vi "Delete_Crossconnection-2.vi"(5 "[IN] Row index\nInitial Point":i32, 7 "[IN] Column in\ndex Initial Point":i32, 9 "[IN] Indicies of Cross\nconnected Points":i32[](array[numeric]), 10 "[IN] The other point \nfor crossconnection found":bool, 11 "[IN] Track group":T1) -> (1 "[OUT] Track group":T1, 2 "[OUT] Column index\nCorrect initial point":i32, 3 "[OUT] Row index\nCorrect initial point":i32)   [LabVIEW 2017]
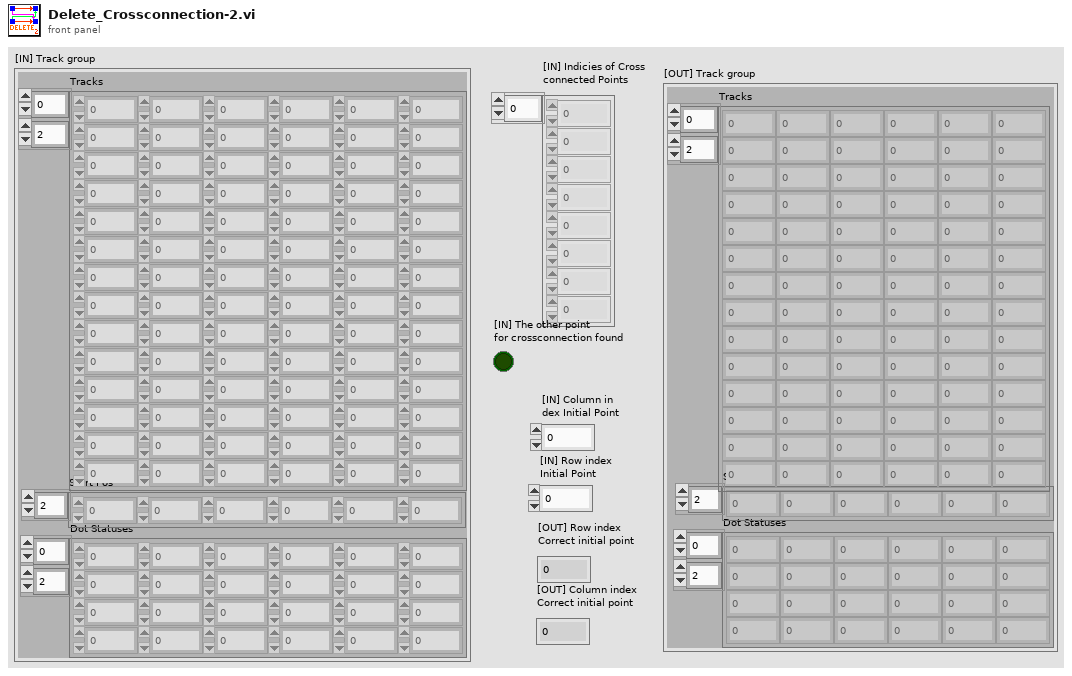
[diagram p1: front panel]
types:
  T1 = cluster{"Tracks":dbl[][], "Start Pos":i32[], "Dot Statuses":i16[][]}
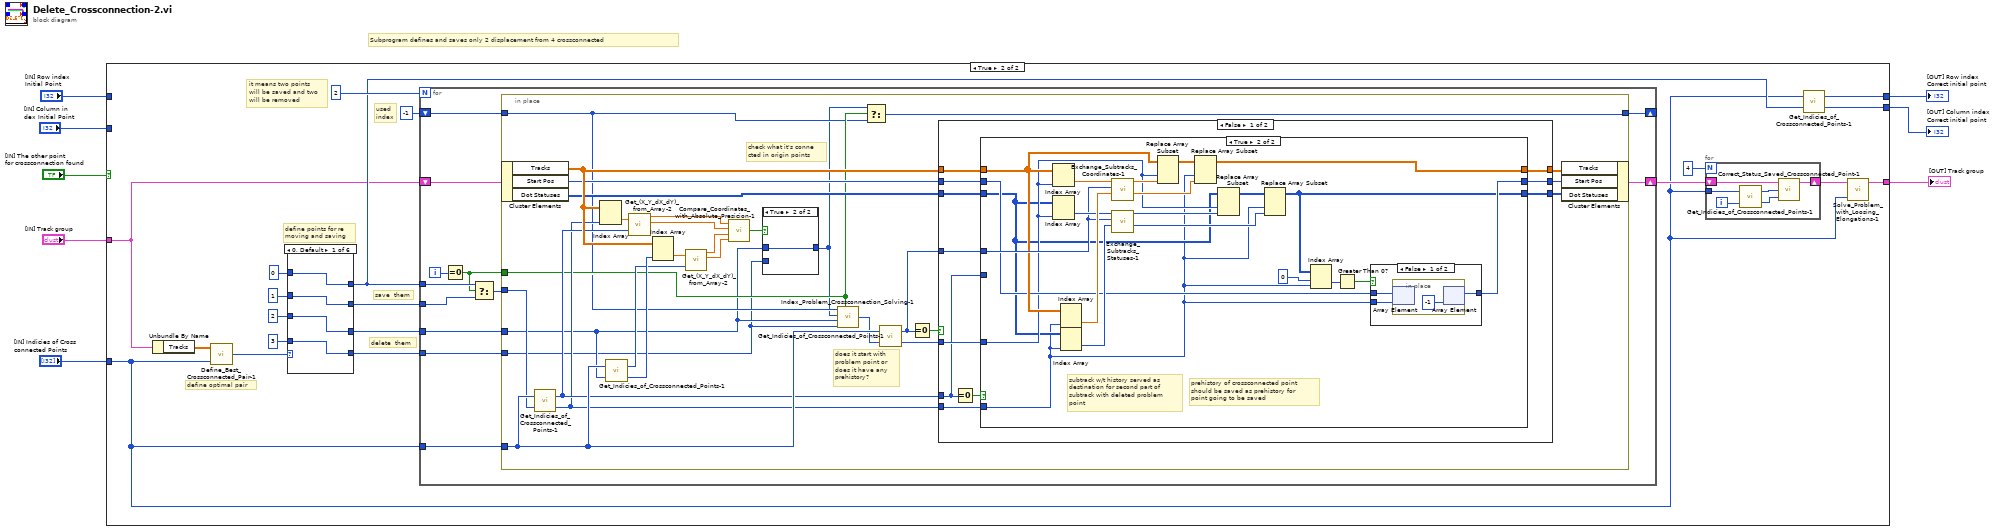
[diagram p0: block diagram]
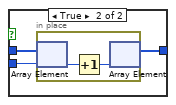
[diagram p4: hidden frame]
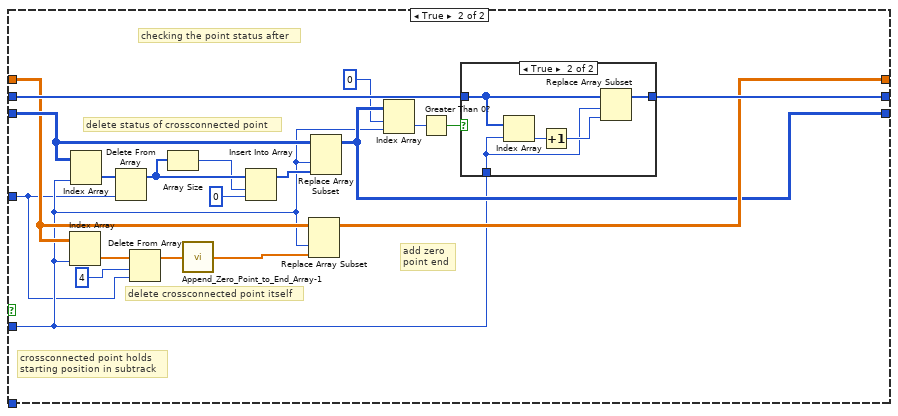
[diagram p5: hidden frame]
diagram:
  # "Subprogram defines and saves only 2 displacement from 4 crossconnected"
  n1 = case shown="True" "[IN] The other point \nfor crossconnection found" {
    tunnel: "[IN] Track group" -> [w11 w19]
    tunnel: "[IN] Indicies of Cross\nconnected Points" -> [_ w13]
    tunnel: [w11 w12] -> w5
    tunnel: [w10 w22] -> w4
    tunnel: [w9 w21] -> w3
    tunnel: "[IN] Row index\nInitial Point" -> [w10 _]
    tunnel: "[IN] Column in\ndex Initial Point" -> [w9 _]
    frame False {
    }
    frame True {
      # "define optimal pair"
      # "used \nindex"
      # "it means two points\nwill be saved and two\nwill be removed"
      # "define points for re\nmoving and saving"
      # "delete  them"
      # "save  them"
      n2 = Unbundle By Name(w19) -> ("Tracks"=w18:dbl[][])
      n3 = call "Define_Best_Crossconnected_Pair-1.vi"("[IN] Indicies of Cross\nconnected Points"=w13, "[IN] Tracks"=w18) -> ("[OUT] Smallest Pair"=w17:i32)  [unwired: 3 in]
      n4 = case shown="0, Default" w17 {
        tunnel: 0 -> [w155 w159 w163 w165 w169 w173]
        tunnel: 1 -> [w154 w157 w161 w167 w171 w172]
        tunnel: 2 -> [w153 w158 w160 w166 w168 w175]
        tunnel: 3 -> [w152 w156 w162 w164 w170 w174]
        tunnel: [w155 w159 w163 w167 w171 w175] -> w23
        tunnel: [w154 w158 w162 w166 w170 w174] -> w24
        tunnel: [w153 w157 w161 w165 w169 w173] -> w27
        tunnel: [w152 w156 w160 w164 w168 w172] -> w26
        frame 0, Default {
        }
        frame 1 {
        }
        frame 2 {
        }
        frame 3 {
        }
        frame 4 {
        }
        frame 5 {
        }
      }
      n5 = for {
        N: 2 -> [_]
        tunnel: w13 -> [w48]
        tunnel: w23 -> [w43]
        tunnel: w24 -> [w42]
        tunnel: w27 -> [w47]
        tunnel: w26 -> [w46]
        shift-right: [w45] -> w15
        shift-left: w19 -> [w49]
        shift-right: [w39] -> _
        shift-left: -1 -> [w40]
        i -> [w44]
        n6 = Equal To 0?(x=w44) -> (x = 0?=w38:bool)
        n7 = Select(t=w43, s=w38, f=w42) -> (s? t:f=w41:i32)
        n8 = in-place {
          in-place-border: w48 -> [w69]
          in-place-border: w47 -> [w51]
          in-place-border: w46 -> [w50]
          in-place-border: w41 -> [w59]
          in-place-border: w40 -> [w54]
          in-place-border: [w56] -> w39
          in-place-border: w38 -> [w55]
          # "does it start with \nproblem point or\ndoes it have any \nprehistory?"
          # "check what it's conne\ncted in origin points"
          n9 = in-place-cluster #1(w49) -> ("Tracks"=w67:dbl[][], "Start Pos"=w66:i32[], "Dot Statuses"=w65:i16[][])
          n10 = call "Get_Indicies_of_Crossconnected_Points-1.vi"("[IN] Index of point"=w59, "[IN] Indicies of Cross\nconnected Points"=w69) -> ("[OUT] Column index"=w57:i32, "[OUT] Row index"=w58:i32)
          n11 = Index Array(array=w67, index (col)=w57) -> (element=w78:dbl[])  [unwired: 1 in]
          n12 = call "Get_Indicies_of_Crossconnected_Points-1.vi"("[IN] Index of point"=w51, "[IN] Indicies of Cross\nconnected Points"=w69) -> ("[OUT] Column index"=w77:i32, "[OUT] Row index"=w75:i32)
          n13 = call "Get_(X_Y_dX_dY)_from_Array-2.vi"("(X,Y,dX,dY)"=w78, "Index of Displacement"=w58) -> ("X"=w74:dbl, "Y"=w73:dbl)  [unwired: 2 out]
          n14 = Index Array(array=w67, index (col)=w77) -> (element=w76:dbl[])  [unwired: 1 in]
          n15 = call "Get_(X_Y_dX_dY)_from_Array-2.vi"("(X,Y,dX,dY)"=w76, "Index of Displacement"=w75) -> ("X"=w72:dbl, "Y"=w71:dbl)  [unwired: 2 out]
          n16 = call "Compare_Coordinates_with_Absolute_Presicion-1.vi"("X 1"=w74, "Y 1"=w73, "X 2"=w72, "Y 2"=w71) -> ("[OUT] Same coordinates?"=w70:bool)  [unwired: 1 in]
          n17 = case shown="True" w70 {
            tunnel: w51 -> [_ w151]
            tunnel: w50 -> [w150 _]
            tunnel: [w150 w151] -> w53
            frame False {
            }
            frame True {
            }
          }
          n18 = call "Index_Problem_Crossconnection_Solving-1.vi"("[IN] Used Index"=w54, "[IN] Defined Index"=w53, "[IN] 1st Index for Deletion"=w51, "[IN] 2nd Index for Deletion"=w50, "[IN] Is it first step?"=w55) -> ("[OUT] Index of Track wi\nth Point For Deletion"=w52:i32)
          n19 = Select(t=w53, s=w55, f=w54) -> (s? t:f=w56:i32)
          n20 = call "Get_Indicies_of_Crossconnected_Points-1.vi"("[IN] Index of point"=w52, "[IN] Indicies of Cross\nconnected Points"=w69) -> ("[OUT] Column index"=w64:i32, "[OUT] Row index"=w62:i32)
          n21 = Equal To 0?(x=w62) -> (x = 0?=w68:bool)
          n22 = case shown="False" w68 {
            tunnel: w67 -> [w88 w133]
            tunnel: w66 -> [w87 w143]
            tunnel: w65 -> [w86 w138]
            tunnel: w64 -> [w81 w128]
            tunnel: [w84 w142] -> w63
            tunnel: w62 -> [w80 w125]
            tunnel: [w85 w131] -> w61
            tunnel: [w83 w129] -> w60
            tunnel: w58 -> [w79 _]
            tunnel: w57 -> [w82 _]
            frame False {
              n23 = Equal To 0?(x=w79) -> (x = 0?=w89:bool)
              n24 = case shown="True" w89 {
                tunnel: w88 -> [w92 w109]
                tunnel: w87 -> [w91 w100]
                tunnel: w86 -> [w90 w97]
                tunnel: [w92 w105] -> w85
                tunnel: [w91 w98] -> w84
                tunnel: [w90 w96] -> w83
                tunnel: w82 -> [_ w95]
                tunnel: w81 -> [_ w99]
                tunnel: w80 -> [_ w110]
                tunnel: w79 -> [_ _]
                frame False {
                  # "I suppose that tracking algorithm will be able to resolve such problem in this case"
                }
                frame True {
                  # "subtrack w/t history served as \ndestination for second part of \nsubtrack with deleted problem \npoint"
                  # "prehistory of crossconnected point \nshould be saved as prehistory for \npoint going to be saved"
                  n25 = Index Array(array=w109, index (col)=w99) -> (element=w114:dbl[])  [unwired: 1 in]
                  n26 = Index Array(array=w97, index (col)=w99) -> (element=w112:i16[])  [unwired: 1 in]
                  n27 = Index Array(array=w109, index (col)=w95) -> (element=w113:dbl[])  [unwired: 1 in]
                  n28 = Index Array(array=w97, index (col)=w95) -> (element=w111:i16[])  [unwired: 1 in]
                  n29 = call "Exchange_Subtracks_Coordinates-1.vi"("[IN] Subtrack wit\nhout prehistory"=w113, "[IN] Row index \nProblem Point"=w110, "[IN] Subtrack \nwith problem"=w114) -> ("[OUT] Reconnected subtrack\n(posthistory after deleted \ncrossconnected point)"=w106:dbl[], "[OUT] Reconnected subtrack\nPrehistory + alternative prob\nlem point"=w108:dbl[])  [unwired: 3 in]
                  n30 = call "Exchange_Subtracks_Statuses-1.vi"("[IN] Statuses wit\nhout prehistory"=w111, "[IN] Row index \nProblem Point"=w110, "[IN] Statuses\nwith problem"=w112) -> ("[OUT] Reconnected statuses\n(posthistory after deleted \ncrossconnected point)"=w102:i16[], "[OUT] Reconnected statuses\nPrehistory + alternative prob\nlem point"=w104:i16[])  [unwired: 3 in]
                  n31 = Replace Array Subset(array=w109, new element=w108, index (col)=w99) -> (w107:dbl[][])  [unwired: 1 in]
                  n32 = Replace Array Subset(array=w107, new element=w106, index (col)=w95) -> (w105:dbl[][])  [unwired: 1 in]
                  n33 = Replace Array Subset(array=w97, new element=w104, index (col)=w99) -> (w103:i16[][])  [unwired: 1 in]
                  n34 = Replace Array Subset(array=w103, new element=w102, index (col)=w95) -> (w96:i16[][])  [unwired: 1 in]
                  n35 = Index Array(array=w96, index (row)=0 ("disabled index (row)"), index (col)=w95) -> (element=w101:i16)
                  n36 = Greater Than 0?(x=w101) -> (x > 0?=w93:bool)
                  n37 = case shown="False" w93 {
                    tunnel: w100 -> [w117 w121]
                    tunnel: w95 -> [w116 w120]
                    tunnel: [w115 w119] -> w98
                    frame False {
                      n38 = in-place {
                        n39 = in-place-array #2(w117, w116) -> ()  [unwired: 1 out]
                        n40 = in-place-array #2(-1) -> (w115:i32[])  [unwired: 1 out]
                      }
                    }
                    frame True {
                      n41 = in-place {
                        n42 = in-place-array #3(w121, w120) -> (w123:i32)
                        n43 = Increment(x=w123) -> (x+1=w122:i32)
                        n44 = in-place-array #3(w122) -> (w119:i32[])  [unwired: 1 out]
                      }
                    }
                  }
                }
              }
            }
            frame True {
              # "add zero \npoint end"
              # "checking the point status after"
              # "delete crossconnected point itself"
              # "delete status of crossconnected point"
              # "crossconnected point holds \nstarting position in subtrack"
              n45 = Index Array(array=w133, index (col)=w128) -> (element=w136:dbl[])  [unwired: 1 in]
              n46 = Index Array(array=w138, index (col)=w128) -> (element=w141:i16[])  [unwired: 1 in]
              n47 = Delete From Array(array=w141, index=w125) -> (array with subset deleted=w140:i16[])  [unwired: 1 in, 1 out]
              n48 = Delete From Array(array=w136, length=4, index=w125) -> (array with subset deleted=w134:dbl[])  [unwired: 1 out]
              n49 = Array Size(array=w140) -> (size(s)=w130:i32)
              n50 = call "Append_Zero_Point_to_End_Array-1.vi"("[IN] Array with \nDisplacements"=w134) -> ("[OUT] Array with \nAppended Point"=w132:dbl[])
              n51 = Insert Into Array(array=w140, index=w130, new element=i16 0 ("new element/subarray")) -> (w137:i16[])
              n52 = Replace Array Subset(array=w133, new element=w132, index (col)=w128) -> (w131:dbl[][])  [unwired: 1 in]
              n53 = Replace Array Subset(array=w138, new element=w137, index (col)=w128) -> (w129:i16[][])  [unwired: 1 in]
              n54 = Index Array(array=w129, index (row)=0 ("disabled index (row)"), index (col)=w128) -> (element=w127:i16)
              n55 = Greater Than 0?(x=w127) -> (x > 0?=w126:bool)
              n56 = case shown="True" w126 {
                tunnel: w143 -> [w144 w149]
                tunnel: [w144 w146] -> w142
                tunnel: w128 -> [_ w145]
                frame False {
                }
                frame True {
                  n57 = Index Array(array=w149, index=w145) -> (element=w148:i32)
                  n58 = Increment(x=w148) -> (x+1=w147:i32)
                  n59 = Replace Array Subset(array=w149, new element=w147, index=w145) -> (w146:i32[])
                }
              }
            }
          }
          n60 = in-place-cluster #1("Tracks"=w61, "Start Pos"=w63, "Dot Statuses"=w60) -> (w45:T1)
        }
      }
      n61 = for {
        N: 4 -> [_]
        shift-right: [w36] -> w14
        shift-left: w15 -> [w37]
        tunnel: w13 -> [w33]
        i -> [w32]
        n62 = call "Get_Indicies_of_Crossconnected_Points-1.vi"("[IN] Index of point"=w32, "[IN] Indicies of Cross\nconnected Points"=w33) -> ("[OUT] Column index"=w34:i32, "[OUT] Row index"=w35:i32)
        n63 = call "Correct_Status_Saved_Crossconnected_Point-1.vi"("[IN] Column index"=w34, "[IN] Row index"=w35, "[IN] Track group"=w37) -> ("[OUT] Track group"=w36:T1)  [unwired: 2 in]
      }
      n64 = call "Get_Indicies_of_Crossconnected_Points-1.vi"("[IN] Index of point"=w23, "[IN] Indicies of Cross\nconnected Points"=w13) -> ("[OUT] Column index"=w21:i32, "[OUT] Row index"=w22:i32)
      n65 = call "Solve_Problem_with_Loosing_Elongations-1.vi"("[IN] Indicies of Cross\nconnected Points"=w13, "[IN] Track group"=w14) -> ("[OUT] Track group"=w12:T1)  [unwired: 3 in]
    }
  }
  "[OUT] Track group" <- w5
  "[OUT] Row index\nCorrect initial point" <- w4
  "[OUT] Column index\nCorrect initial point" <- w3
